vi "Stop Core.vi"(10 "final error code":i32, 11 "Evaporative Cooler":refnum<class "Evaporative Cooler.lvclass">) -> (3 "Evaporative Cooler":refnum<class "Evaporative Cooler.lvclass">)   [LabVIEW 2025, in "Evaporative Cooler.lvlib" / "Evaporative Cooler.lvclass"]
doc: "In override VIs of Stop Core.vi, an actor should invoke any code needed to stop all the parallel processes that it created during its run. This includes any nested actors that it created and any other asynchronously running VIs, such as a Time-Delayed Message. It may also include all parallel loops in its Actor Core, although it is acceptable to stop those using a local signal on the Actor Core block diagram that is raised after the Call Parent Node finishes. \n\nThe <b>final error code</b> input tells the actor what error was set when this actor quit. Zero means there was no error. You can use this to decide whether this should be treated as a Normal Stop or an Emergency Stop for the purposes of signaling other actors. In general, any non-zero value should be treated as an Emergency Stop, though a given actor is free to choose other policies. Note that the particular error code 1608 indicates that this actor was itself stopped by an Emergency Stop and should pass that along."
uses:
  Evaporative Cooler.lvclass
  <vilib>/ActorFramework/Time-Delayed Send Message/Time-Delay Override Options.ctl
  Evaporative Cooler.lvclass/Evaporative Cooler.ctl
  <vilib>/ActorFramework/Stop Msg/Stop Msg.lvclass/Stop Msg.ctl
  <vilib>/ActorFramework/Message Enqueuer/Message Enqueuer.lvclass/Message Enqueuer.ctl
  <vilib>/ActorFramework/Stop Msg/Send Emergency Stop.vi
  <vilib>/ActorFramework/Stop Msg/Send Normal Stop.vi
  <vilib>/ActorFramework/Message Enqueuer/Enqueue Critical.vi
  <vilib>/ActorFramework/Message Enqueuer/Enqueue.vi
  <vilib>/ActorFramework/Stop Msg/Stop Msg.lvclass
  C:/Program Files/National Instruments/LabVIEW 2025/vi.lib/ActorFramework/Message/Message.lvclass
  <vilib>/ActorFramework/Message Priority Queue/Priority Enqueue.vi
  Cooler/Cooler/Cooler.lvclass
  <vilib>/ActorFramework/Actor Framework.lvlib
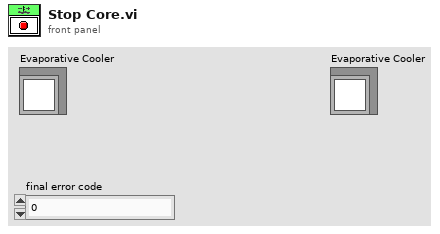
[diagram p1: front panel]
types:
  T1 = typedef "Actor Framework.lvlib/Time-Delay Override Options.ctl" = enum16{"Send next copy now", "Skip next scheduled copy", "Send next copy now and stop all further copies", "Stop all further copies"}
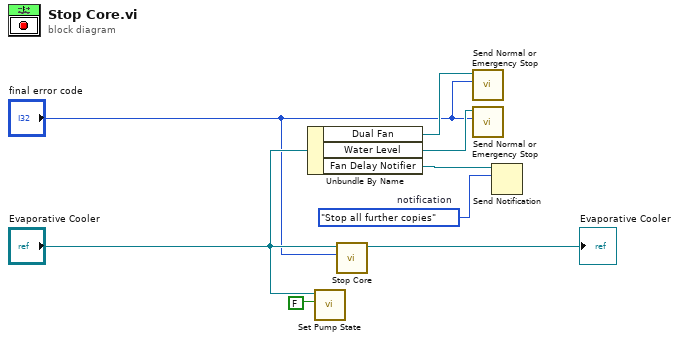
[diagram p0: block diagram]
diagram:
  w7 = Time-Delay_Override_Options."Stop all further copies"  # notification
  n1 = Unbundle By Name("Evaporative Cooler") -> ("Dual Fan"=w3:refnum<class "Message Enqueuer.lvclass">, "Water Level"=w2:refnum<class "Message Enqueuer.lvclass">, "Fan Delay Notifier"=w6:refnum<notifier>)
  n2 = call-dynamic "Set Pump State.vi"("Pump State"=FALSE, "Evaporative Cooler in"="Evaporative Cooler") -> ()  [unwired: 9 in, 1 out]
  n3 = call-parent "Stop Core.vi"("final error code"="final error code", "Actor in"="Evaporative Cooler") -> ("Actor out"=→"Evaporative Cooler":refnum<class "Evaporative Cooler.lvclass">)  [unwired: 9 in]
  n4 = call <vilib>:"Send Normal or Emergency Stop.vi"("final error code"="final error code", "Message Enqueuer"=w3) -> ()  [unwired: 9 in, 1 out]
  n5 = call <vilib>:"Send Normal or Emergency Stop.vi"("final error code"="final error code", "Message Enqueuer"=w2) -> ()  [unwired: 9 in, 1 out]
  n6 = Send Notification(notification=w7, notifier=w6) -> ()  [unwired: 1 in, 2 out]
